vi "DataToXML.vi"(8 "error in":errorcluster, 11 "path":path) -> (0 "error out":errorcluster, 3 "XML":string)   [LabVIEW 2013, in "main.lvlib"]
uses:
  main.lvlib
  <vilib>/xml/Close Reference(Node).vi
  <vilib>/xml/NI_XML.lvlib
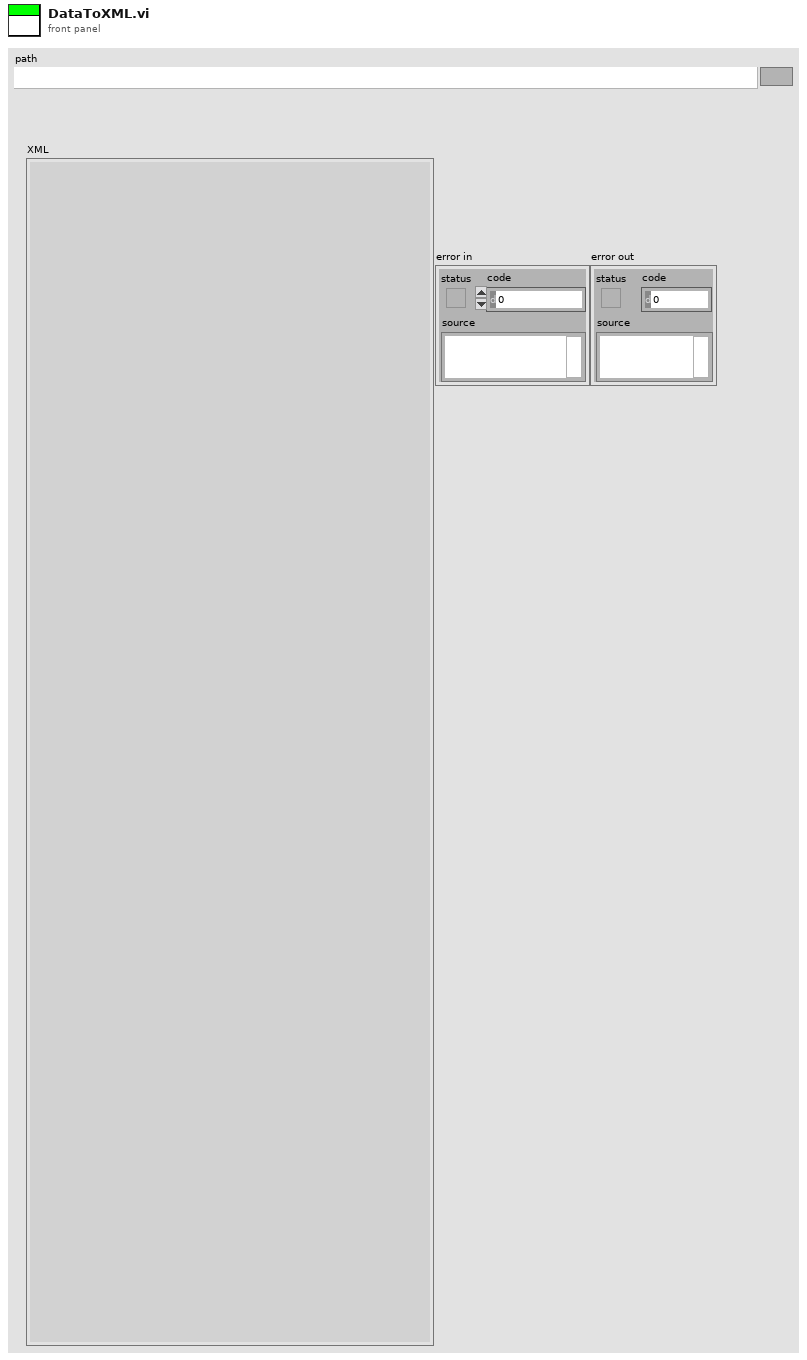
[diagram p1: front panel]
types:
  T1 = cluster{"sys":dbl, "dia":dbl, "puls":dbl, "date":string, "time":string, "code":string, "serial":string, "temp":dbl, "activity":string}[]
  T2 = cluster{"Palpation":string[], "Personal Info":string[], "Hospital":string[]}
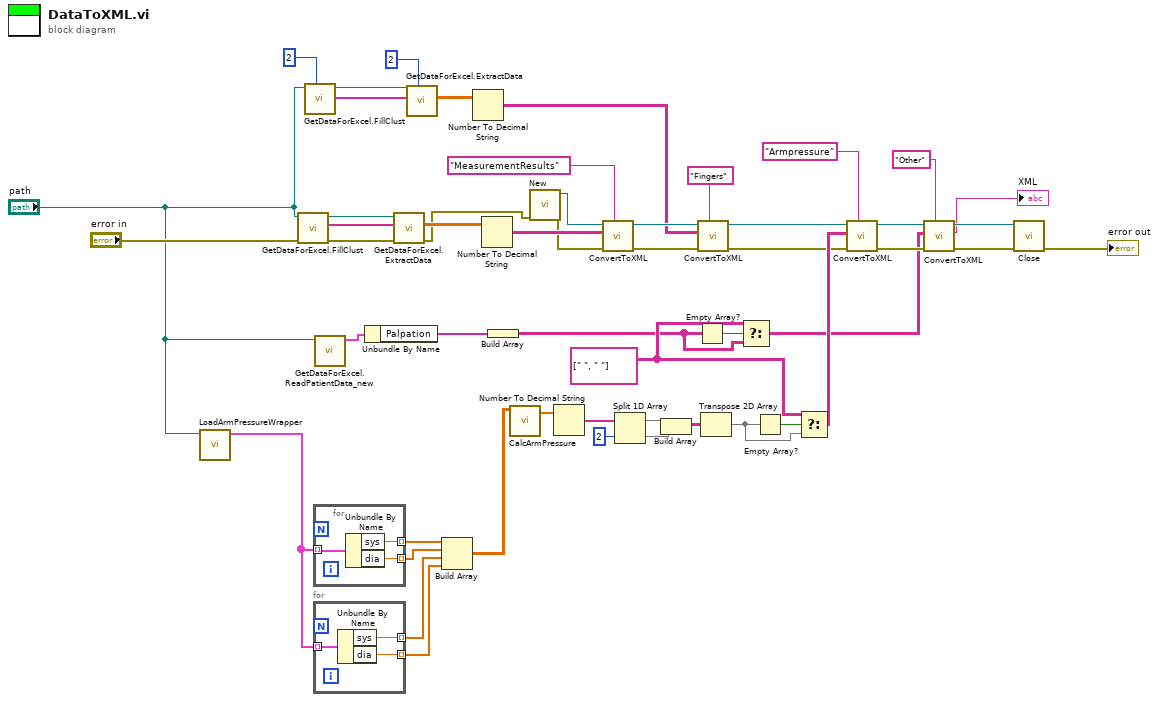
[diagram p0: block diagram]
diagram:
  w23 = string[][] [[" ", " "]] ("DataInput")
  n1 = call "LoadArmPressureWrapper.vi"("File dir"="path") -> ("Armpressure Right"=w6:T1)  [unwired: 8 in, 2 out]
  n2 = call "GetDataForExcel.FillClust.vi"("error in"="error in", "path"="path") -> ("error out"=w50:errorcluster, "Array"=w49:string[], "path out"=w51:path)  [unwired: 7 in]
  n3 = call "GetDataForExcel.FillClust.vi"("Type"=u16 2 ("Numeric"), "path"="path") -> ("Array"=w19:string[], "path out"=w20:path)  [unwired: 7 in, 1 out]
  n4 = for {
    tunnel: w6 -> [w54] mode=indexing
    tunnel: [w53] -> w5 mode=indexing
    tunnel: [w52] -> w4 mode=indexing
    n5 = Unbundle By Name(w54) -> ("sys"=w53:dbl, "dia"=w52:dbl)
  }
  n6 = for {
    tunnel: w6 -> [w57] mode=indexing
    tunnel: [w56] -> w3 mode=indexing
    tunnel: [w55] -> w2 mode=indexing
    n7 = Unbundle By Name(w57) -> ("sys"=w56:dbl, "dia"=w55:dbl)
  }
  n8 = call "GetDataForExcel.ReadPatientData_new.vi"("Path"="path") -> ("output cluster"=w11:T2)  [unwired: 9 in, 1 out]
  n9 = Unbundle By Name(w11) -> ("Palpation"=w10:string[])
  n10 = call "GetDataForExcel.ExtractData.vi"("Error In"=w50, "Folders"=w49, "Path"=w51) -> ("Error Out"=w31:errorcluster, "Data"=w48:dbl[][])  [unwired: 6 in, 1 out]
  n11 = call "GetDataForExcel.ExtractData.vi"("Report Type"=2, "Folders"=w19, "Path"=w20) -> ("Data"=w13:dbl[][])  [unwired: 6 in, 2 out]
  n12 = Build Array(w5, w4, w3, w2) -> (w1:dbl[][])
  n13 = Number To Decimal String(number=w13) -> (decimal integer string=w12:string[][])  [unwired: 1 in]
  n14 = Number To Decimal String(number=w48) -> (decimal integer string=w47:string[][])  [unwired: 1 in]
  n15 = Build Array(w10) -> (w9:string[][])
  n16 = call "CalcArmPressure.vi"("Armpres"=w1) -> ("Array Out"=w42:dbl[])  [unwired: 8 in, 2 out]
  n17 = call <vilib>:"New.vi"("error in (no error)"=w31) -> ("error out"=w44:errorcluster, "DOM document out"=w45:refnum<k20>)  [unwired: 7 in]
  n18 = Number To Decimal String(number=w42) -> (decimal integer string=w41:string[])  [unwired: 1 in]
  n19 = call "ConvertToXML.vi"("InputTag"="MeasurementResults" ("Tag Name"), "error in (no error)"=w44, "DataInput"=w47, "DOM document in"=w45) -> ("error out"=w21:errorcluster, "DOM document out"=w22:refnum<k20>)  [unwired: 5 in, 1 out]
  n20 = Split 1D Array(array=w41, index=2) -> (first subarray=w39:string[], second subarray=w38:string[])
  n21 = Build Array(w39, w38) -> (w28:string[][])
  n22 = Empty Array?(array=w9) -> (empty?=w24:bool)
  n23 = call "ConvertToXML.vi"("InputTag"="Fingers", "error in (no error)"=w21, "DataInput"=w12, "DOM document in"=w22) -> ("error out"=w16:errorcluster, "DOM document out"=w15:refnum<k20>)  [unwired: 5 in, 1 out]
  n24 = Transpose 2D Array(2D array=w28) -> (transposed array=w26:string[][])
  n25 = Select(t=w23, s=w24, f=w9) -> (s? t:f=w8:string[][])
  n26 = Empty Array?(array=w26) -> (empty?=w27:bool)
  n27 = Select(t=w23, s=w27, f=w26) -> (s? t:f=w25:string[][])
  n28 = call "ConvertToXML.vi"("InputTag"="Armpressure", "error in (no error)"=w16, "DataInput"=w25, "DOM document in"=w15) -> ("error out"=w36:errorcluster, "DOM document out"=w37:refnum<k20>)  [unwired: 5 in, 1 out]
  n29 = call "ConvertToXML.vi"("InputTag"="Other", "error in (no error)"=w36, "DataInput"=w8, "DOM document in"=w37) -> ("error out"=w33:errorcluster, "XML"=→"XML":string, "DOM document out"=w34:refnum<k20>)  [unwired: 5 in]
  n30 = call-poly <vilib>:"Close.vi"("error in (no error)"=w33, "node"=w34) -> ("error out"=→"error out":errorcluster)  [unwired: 7 in]
